vi "Clamp.vi"(8 "error in (no error)":errorcluster, 11 "Instrument.Oxford1820 in":refnum<class "Instrument.Oxford1820.lvclass">) -> (0 "error out":errorcluster, 3 "Instrument.Oxford1820 out":refnum<class "Instrument.Oxford1820.lvclass">)   [LabVIEW 2016, in "Instrument.Oxford1820.lvclass"]
uses:
  Instrument.Oxford1820.lvclass
  <instrlib>/Mercury iXX/Public/Libraries/Magnet/Controls/PSU Actions.ctl
  Typedefs/Instrument.Oxford1820.Commands-enum.ctl
  <instrlib>/Mercury iXX/Public/Libraries/Magnet.lvlib
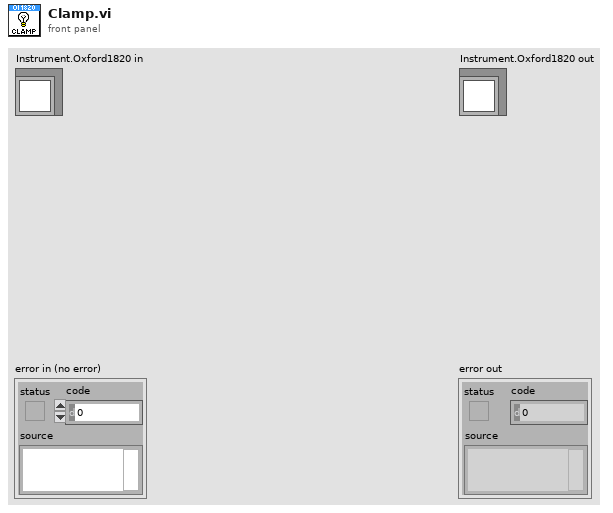
[diagram p1: front panel]
types:
  T1 = typedef "Instrument.Oxford1820.lvclass/Instrument.Oxford1820.Commands-enum.ctl" = enum16{"setAction", "setTarget", "setSwitchHeat", "setLambda", "setFillMode", "setNeedleValve", "setMagnetField", "getStatus", "getTarget", "getSwitchHeat", "getPSUField", "getMagnetField"}
  T2 = typedef "Mercury iXX.lvlib/Magnet.lvlib/PSU Actions.ctl" = string
  T3 = cluster{"Hold":bool, "Ramp to Setpoint":bool, "Ramp to Zero":bool, "Clamp":bool}
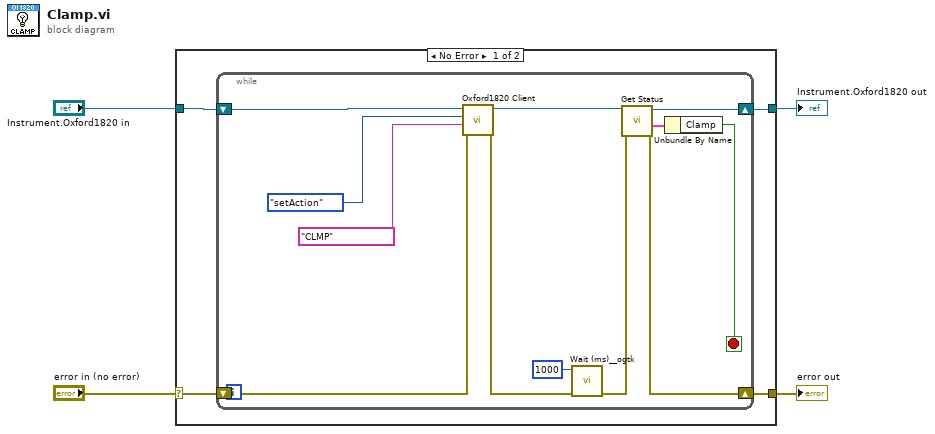
[diagram p0: block diagram]
diagram:
  n1 = case shown="No Error" "error in (no error)" {
    selector: "error in (no error)" -> [w7 w22]
    tunnel: [w5 w22] -> w3
    tunnel: [w6 w21] -> w1
    tunnel: "Instrument.Oxford1820 in" -> [w8 w21]
    frame No Error {
      n2 = while {
        shift-right: [w13] -> w6
        shift-left: w8 -> [w18]
        shift-right: [w10] -> w5
        shift-left: w7 -> [w17]
        stop <- w9 stop-if-true
        n3 = call "Oxford1820 Client.vi"("error in (no error)"=w17, "Data"=T2 "CLMP" ("PSU Act Stat"), "Commands"=Instrument.Oxford1820.Commands-enum."setAction", "Instrument.1820 in"=w18) -> ("error out"=w11:errorcluster, "Instrument.1820 out"=w14:refnum<class "Instrument.Oxford1820.lvclass">)  [unwired: 5 in, 1 out]
        n4 = call <userlib>:"Wait (ms)__ogtk.vi"("error in (no error)"=w11, "milliseconds to wait"=u32 1000) -> ("error out"=w12:errorcluster)  [unwired: 8 in, 1 out]
        n5 = call-dynamic "Get Status.vi"("error in (no error)"=w12, "Instrument.Oxford1820 in"=w14) -> ("error out"=w10:errorcluster, "Status"=w15:T3, "Instrument.Oxford1820 out"=w13:refnum<class "Instrument.Oxford1820.lvclass">)  [unwired: 6 in, 1 out]
        n6 = Unbundle By Name(w15) -> ("Clamp"=w9:bool)
      }
    }
    frame Error {
    }
  }
  "error out" <- w3
  "Instrument.Oxford1820 out" <- w1
